vi "GVSView Form Title Frame.vi"() -> ()   [LabVIEW 2013]
uses:
  <vilib>/Utility/miscctls.llb/LVPointTypeDef.ctl
  <vilib>/Utility/miscctls.llb/LVBoundsTypeDef.ctl
  <vilib>/Utility/miscctls.llb/LVPositionTypeDef.ctl
  SubVI/GVSMain Sub Window Global.vi
  GVSView Global.vi
panel:
  in  "pSPRefParent":refnum<vi>
  in  "sClickState":string
  in  "nActiveState":i32
  in  "nIDFrame":i32
  in  "IconRing":u16(ring)
  in  "sViewName":string
  out "TitleName":string caption="Title Name"
  in  "StateOut":bool
  in  "stop":bool
  in  "InActiveClose":bool
  in  "ActiveClose":bool
  in  "bSPResize":bool
  in  "InActiveState":bool
  in  "ActiveStateHalf":bool
  out "SubVI Ref":refnum<vi>
  in  "ActiveState":bool
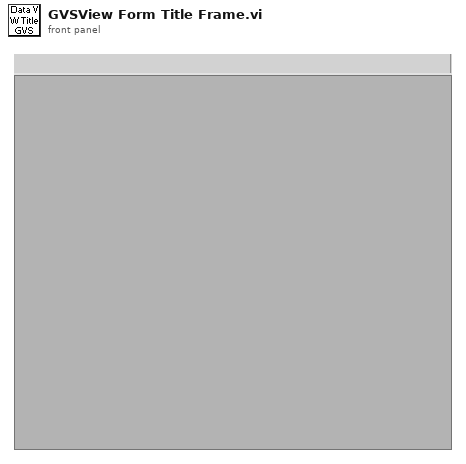
[diagram p1: front panel]
types:
  T1 = typedef "LVPointTypeDef.ctl" = cluster{"Horizontal":i16, "Vertical":i16}
  T2 = typedef "LVBoundsTypeDef.ctl" = cluster{"Width":u32, "Height":u32}
  T3 = typedef "LVPositionTypeDef.ctl" = cluster{"Left":i32, "Top":i32}
  T4 = typedef "LVRectTypeDef.ctl" = cluster{"Left":i16, "Top":i16, "Right":i16, "Bottom":i16}
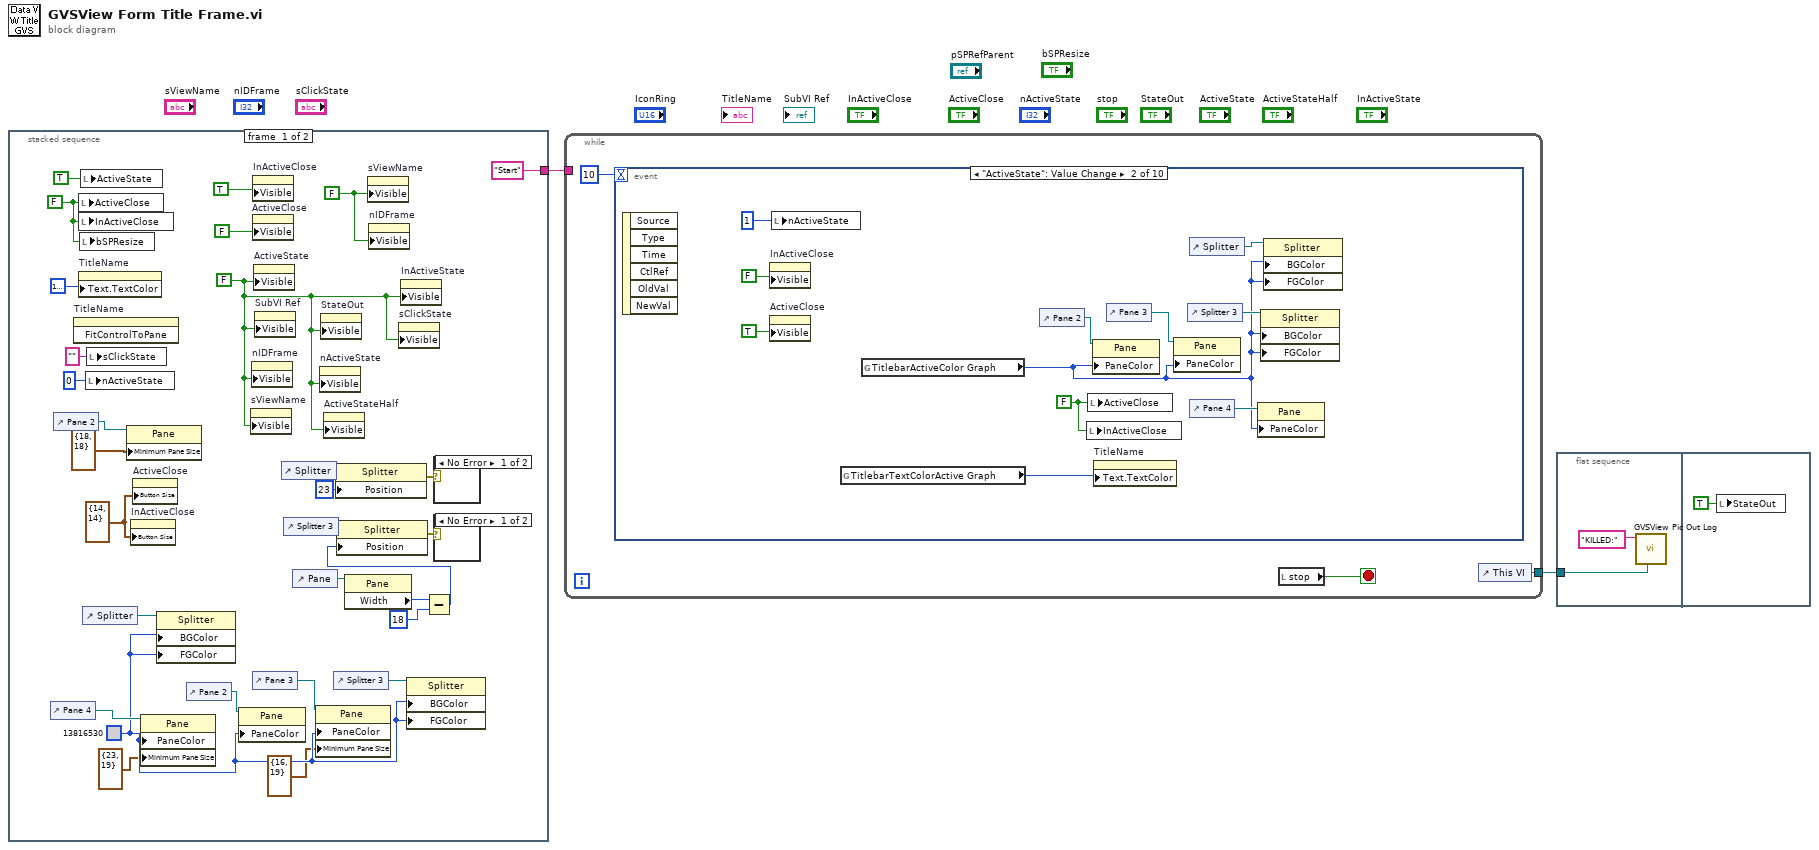
[diagram p0: block diagram]
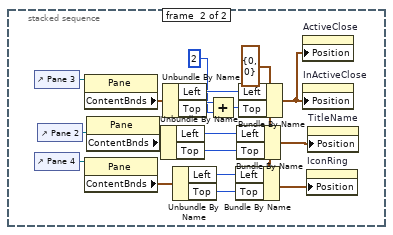
[diagram p4: hidden frame]
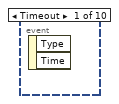
[diagram p5: hidden frame]
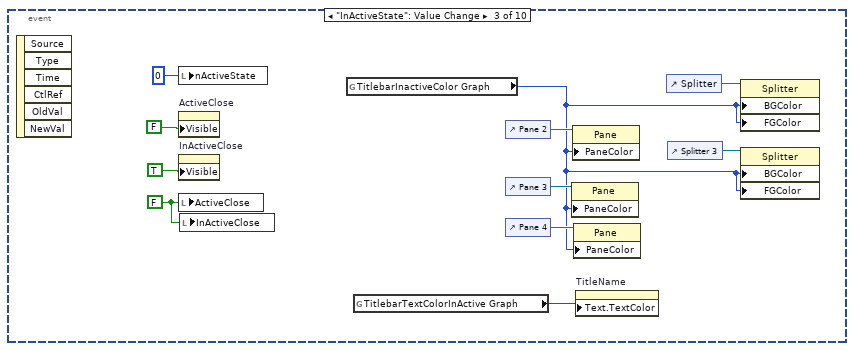
[diagram p6: hidden frame]
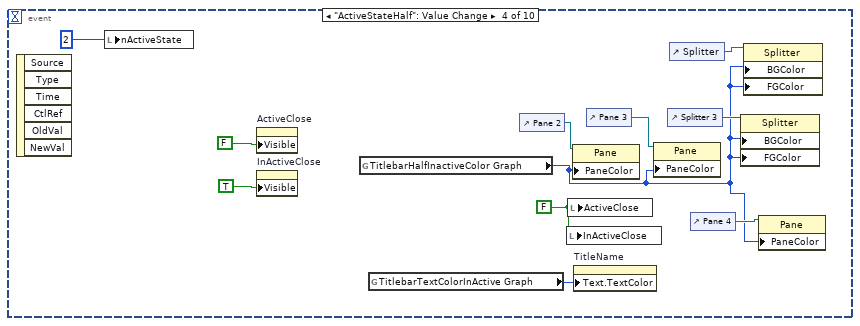
[diagram p7: hidden frame]
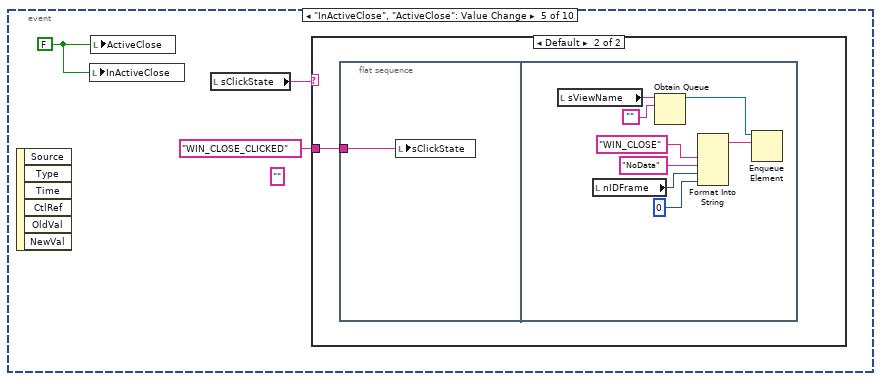
[diagram p8: hidden frame]
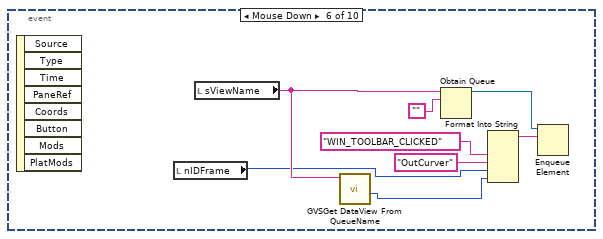
[diagram p10: hidden frame]
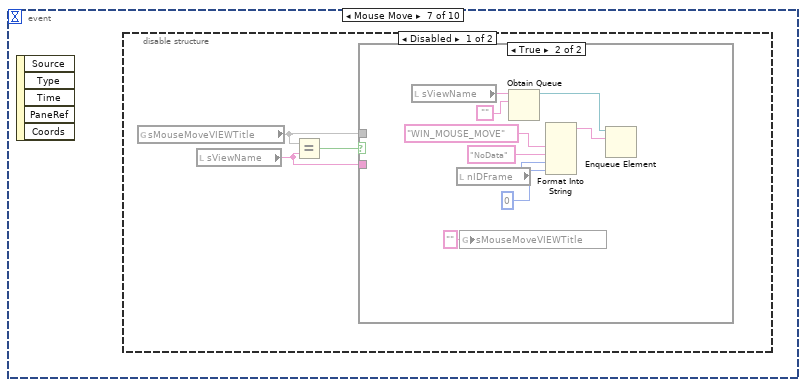
[diagram p11: hidden frame]
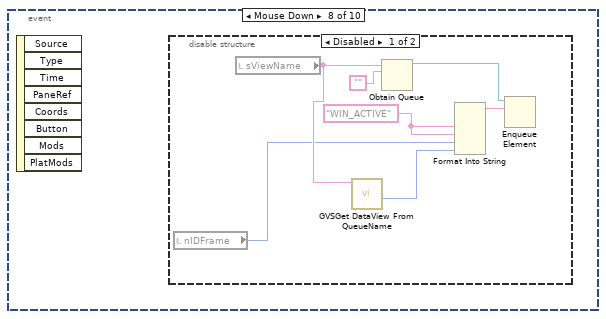
[diagram p14: hidden frame]
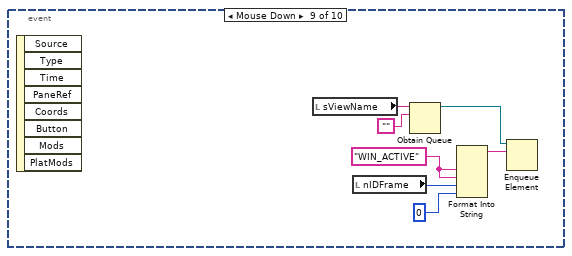
[diagram p16: hidden frame]
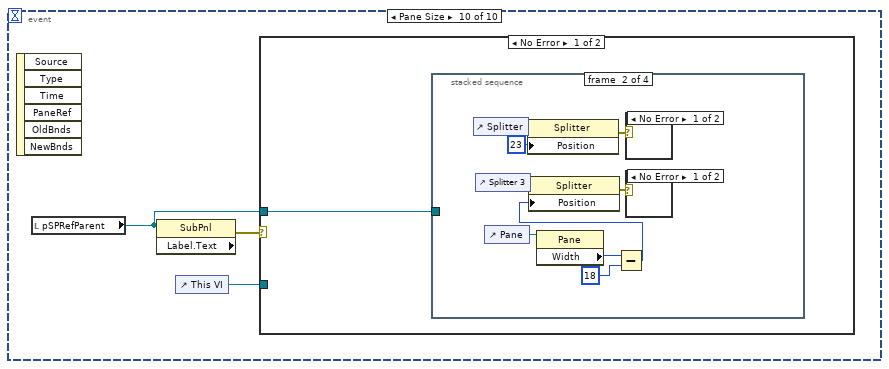
[diagram p17: hidden frame]
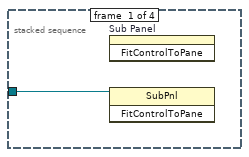
[diagram p18: hidden frame]
diagram:
  n1 = stacked-sequence {
    tunnel: ["Start" _] -> w1
    frame #0 {
      w19 = FALSE ("ToolBar Click")
      w21 = T2 {"Width"=14, "Height"=14} ("Button Size")
      w17 = FALSE ("ToolBar Click")
      w22 = u32 13816530
      w14 = FALSE ("Stop")
      n2 = control-ref of="Pane 4"() -> (w24:refnum<vi>)
      n3 = control-ref of="Pane 2"() -> (w26:refnum<vi>)
      n4 = invoke on="TitleName" class="Str" method="FitControlToPane"() -> ()  [unwired: 3 in, 3 out]
      n5 = local write "ActiveClose"(w14) -> ()
      n6 = local write "InActiveClose"(w14) -> ()
      n7 = property on="TitleName" class="Str"("Text.TextColor"=u32 16777222) -> ()  [unwired: 2 in, 2 out]
      n8 = local write "bSPResize"(w14) -> ()
      n9 = local write "ActiveState"(TRUE ("ActiveState")) -> ()
      n10 = control-ref of="Splitter"() -> (w23:refnum<vi>)
      n11 = local write "nActiveState"(0) -> ()
      n12 = local write "sClickState"("" ("sClickState")) -> ()
      n13 = property class="Pane"(reference=w26, "Minimum Pane Size"=T1 {"Horizontal"=18, "Vertical"=18}) -> ()  [unwired: 1 in, 2 out]
      n14 = property on="InActiveClose" class="Bool (strict)"("Button Size"=w21) -> ()  [unwired: 2 in, 2 out]
      n15 = property on="ActiveClose" class="Bool (strict)"("Button Size"=w21) -> ()  [unwired: 2 in, 2 out]
      n16 = property class="Pane"(reference=w24, "PaneColor"=w22, "Minimum Pane Size"=T1 {"Horizontal"=23, "Vertical"=19}) -> ()  [unwired: 1 in, 2 out]
      n17 = property class="Splitter"(reference=w23, "BGColor"=w22, "FGColor"=w22) -> ()  [unwired: 1 in, 2 out]
      n18 = control-ref of="Pane 2"() -> (w25:refnum<vi>)
      n19 = property class="Pane"(reference=w25, "PaneColor"=w22) -> ()  [unwired: 1 in, 2 out]
      n20 = property on="sViewName" class="Str"("Visible"=w17) -> ()  [unwired: 2 in, 2 out]
      n21 = property on="nIDFrame" class="DigNum (strict)"("Visible"=w17) -> ()  [unwired: 2 in, 2 out]
      n22 = property on="InActiveClose" class="Bool (strict)"("Visible"=TRUE ("ToolBar Click")) -> ()  [unwired: 2 in, 2 out]
      n23 = property on="ActiveClose" class="Bool (strict)"("Visible"=FALSE ("ToolBar Click")) -> ()  [unwired: 2 in, 2 out]
      n24 = control-ref of="Pane 3"() -> (w31:refnum<vi>)
      n25 = property on="ActiveState" class="Bool (strict)"("Visible"=w17) -> ()  [unwired: 2 in, 2 out]
      n26 = property on="SubVI Ref" class="VIRef (strict)"("Visible"=w17) -> ()  [unwired: 2 in, 2 out]
      n27 = control-ref of="Splitter"() -> (w5:refnum<vi>)
      n28 = control-ref of="Splitter 3"() -> (w6:refnum<vi>)
      n29 = control-ref of="Pane"() -> (w8:refnum<vi>)
      n30 = property class="Pane"(reference=w31, "PaneColor"=w22, "Minimum Pane Size"=T1 {"Horizontal"=16, "Vertical"=19}) -> ()  [unwired: 1 in, 2 out]
      n31 = property on="nActiveState" class="DigNum (strict)"("Visible"=w17) -> ()  [unwired: 2 in, 2 out]
      n32 = property on="StateOut" class="Bool (strict)"("Visible"=w17) -> ()  [unwired: 2 in, 2 out]
      n33 = property on="ActiveStateHalf" class="Bool (strict)"("Visible"=w17) -> ()  [unwired: 2 in, 2 out]
      n34 = control-ref of="Splitter 3"() -> (w30:refnum<vi>)
      n35 = property class="Splitter"(reference=w5, "Position"=23 ("Splitter Position")) -> (error out=w11:errorcluster)  [unwired: 1 in, 1 out]
      n36 = property class="Pane"(reference=w8) -> ("Width"=w9:u32)  [unwired: 1 in, 2 out]
      n37 = property on="sViewName" class="Str"("Visible"=w19) -> ()  [unwired: 2 in, 2 out]
      n38 = property on="nIDFrame" class="DigNum (strict)"("Visible"=w19) -> ()  [unwired: 2 in, 2 out]
      n39 = property on="sClickState" class="Str"("Visible"=w17) -> ()  [unwired: 2 in, 2 out]
      n40 = property on="InActiveState" class="Bool (strict)"("Visible"=w17) -> ()  [unwired: 2 in, 2 out]
      n41 = property class="Splitter"(reference=w30, "BGColor"=w22, "FGColor"=w22) -> ()  [unwired: 1 in, 2 out]
      n42 = Subtract(x=w9, y=u32 18) -> (x-y=w10:u32)
      n43 = property class="Splitter"(reference=w6, "Position"=w10) -> (error out=w12:errorcluster)  [unwired: 1 in, 1 out]
      n44 = case shown="No Error" w11 {
        frame No Error {
        }
        frame Error {
        }
      }
      n45 = case shown="No Error" w12 {
        frame No Error {
        }
        frame Error {
        }
      }
    }
    frame #1 {
      w50 = T3 {"Left"=0, "Top"=0} ("Position")
      n46 = control-ref of="Pane 3"() -> (w40:refnum<vi>)
      n47 = control-ref of="Pane 4"() -> (w48:refnum<vi>)
      n48 = control-ref of="Pane 2"() -> (w33:refnum<vi>)
      n49 = property class="Pane"(reference=w40) -> ("ContentBnds"=w39:T4)  [unwired: 1 in, 2 out]
      n50 = property class="Pane"(reference=w48) -> ("ContentBnds"=w46:T4)  [unwired: 1 in, 2 out]
      n51 = property class="Pane"(reference=w33) -> ("ContentBnds"=w43:T4)  [unwired: 1 in, 2 out]
      n52 = Unbundle By Name(w43) -> ("Left"=w42:i16, "Top"=w44:i16)
      n53 = Unbundle By Name(w39) -> ("Left"=w38:i16, "Top"=w36:i16)
      n54 = Unbundle By Name(w46) -> ("Left"=w47:i16, "Top"=w45:i16)
      n55 = Add(x=w36, y=i16 2) -> (x+y=w37:i16)
      n56 = Bundle By Name(cluster=w50, "Left"=w47, "Top"=w45) -> (w49:T3)
      n57 = Bundle By Name(cluster=w50, "Left"=w42, "Top"=w44) -> (w41:T3)
      n58 = Bundle By Name(cluster=w50, "Left"=w38, "Top"=w37) -> (w34:T3)
      n59 = property on="ActiveClose" class="Bool (strict)"("Position"=w34) -> ()  [unwired: 2 in, 2 out]
      n60 = property on="InActiveClose" class="Bool (strict)"("Position"=w34) -> ()  [unwired: 2 in, 2 out]
      n61 = property on="IconRing" class="Ring (strict)"("Position"=w49) -> ()  [unwired: 2 in, 2 out]
      n62 = property on="TitleName" class="Str"("Position"=w41) -> ()  [unwired: 2 in, 2 out]
    }
  }
  n63 = while {
    tunnel: [w52] -> w2
    tunnel: w1 -> [_]
    stop <- w51 stop-if-true
    n64 = event shown="[1] \"ActiveState\": Value Change" {
      selector: _ -> [_ _ _ _ _ _ _ _ _ _]
      dyn-events: _ -> [_ _ _ _ _ _ _ _ _ _]
      timeout: 10 -> [_ _ _ _ _ _ _ _ _ _]
      event Timeout {
        n65 = event-data() -> ()  [unwired: 3 out]
      }
      event "ActiveState": Value Change {
        w62 = FALSE ("Stop")
        n66 = event-data() -> ()  [unwired: 7 out]
        n67 = property on="InActiveClose" class="Bool (strict)"("Visible"=FALSE ("ToolBar Click")) -> ()  [unwired: 2 in, 2 out]
        n68 = property on="ActiveClose" class="Bool (strict)"("Visible"=TRUE ("ToolBar Click")) -> ()  [unwired: 2 in, 2 out]
        n69 = local write "nActiveState"(1) -> ()
        n70 = global read "GVSMain Sub Window Global.vi" "TitlebarTextColorActive Graph"() -> (w55:u32)
        n71 = global read "GVSMain Sub Window Global.vi" "TitlebarActiveColor Graph"() -> (w54:u32)
        n72 = control-ref of="Pane 2"() -> (w61:refnum<vi>)
        n73 = local write "InActiveClose"(w62) -> ()
        n74 = local write "ActiveClose"(w62) -> ()
        n75 = property class="Pane"(reference=w61, "PaneColor"=w54) -> ()  [unwired: 1 in, 2 out]
        n76 = property on="TitleName" class="Str"("Text.TextColor"=w55) -> ()  [unwired: 2 in, 2 out]
        n77 = control-ref of="Pane 3"() -> (w64:refnum<vi>)
        n78 = property class="Pane"(reference=w64, "PaneColor"=w54) -> ()  [unwired: 1 in, 2 out]
        n79 = control-ref of="Splitter 3"() -> (w63:refnum<vi>)
        n80 = control-ref of="Splitter"() -> (w59:refnum<vi>)
        n81 = control-ref of="Pane 4"() -> (w60:refnum<vi>)
        n82 = property class="Pane"(reference=w60, "PaneColor"=w54) -> ()  [unwired: 1 in, 2 out]
        n83 = property class="Splitter"(reference=w63, "BGColor"=w54, "FGColor"=w54) -> ()  [unwired: 1 in, 2 out]
        n84 = property class="Splitter"(reference=w59, "BGColor"=w54, "FGColor"=w54) -> ()  [unwired: 1 in, 2 out]
      }
      event "InActiveState": Value Change {
        w73 = FALSE ("Stop")
        n85 = event-data() -> ()  [unwired: 7 out]
        n86 = local write "nActiveState"(0) -> ()
        n87 = property on="ActiveClose" class="Bool (strict)"("Visible"=FALSE ("ToolBar Click")) -> ()  [unwired: 2 in, 2 out]
        n88 = property on="InActiveClose" class="Bool (strict)"("Visible"=TRUE ("ToolBar Click")) -> ()  [unwired: 2 in, 2 out]
        n89 = local write "ActiveClose"(w73) -> ()
        n90 = local write "InActiveClose"(w73) -> ()
        n91 = global read "GVSMain Sub Window Global.vi" "TitlebarInactiveColor Graph"() -> (w65:u32)
        n92 = global read "GVSMain Sub Window Global.vi" "TitlebarTextColorInActive Graph"() -> (w66:u32)
        n93 = control-ref of="Pane 2"() -> (w72:refnum<vi>)
        n94 = control-ref of="Pane 3"() -> (w75:refnum<vi>)
        n95 = control-ref of="Pane 4"() -> (w71:refnum<vi>)
        n96 = property class="Pane"(reference=w75, "PaneColor"=w65) -> ()  [unwired: 1 in, 2 out]
        n97 = property class="Pane"(reference=w72, "PaneColor"=w65) -> ()  [unwired: 1 in, 2 out]
        n98 = property class="Pane"(reference=w71, "PaneColor"=w65) -> ()  [unwired: 1 in, 2 out]
        n99 = property on="TitleName" class="Str"("Text.TextColor"=w66) -> ()  [unwired: 2 in, 2 out]
        n100 = control-ref of="Splitter"() -> (w70:refnum<vi>)
        n101 = control-ref of="Splitter 3"() -> (w74:refnum<vi>)
        n102 = property class="Splitter"(reference=w70, "BGColor"=w65, "FGColor"=w65) -> ()  [unwired: 1 in, 2 out]
        n103 = property class="Splitter"(reference=w74, "BGColor"=w65, "FGColor"=w65) -> ()  [unwired: 1 in, 2 out]
      }
      event "ActiveStateHalf": Value Change {
        w84 = FALSE ("Stop")
        n104 = event-data() -> ()  [unwired: 7 out]
        n105 = local write "nActiveState"(2) -> ()
        n106 = property on="ActiveClose" class="Bool (strict)"("Visible"=FALSE ("ToolBar Click")) -> ()  [unwired: 2 in, 2 out]
        n107 = property on="InActiveClose" class="Bool (strict)"("Visible"=TRUE ("ToolBar Click")) -> ()  [unwired: 2 in, 2 out]
        n108 = global read "GVSMain Sub Window Global.vi" "TitlebarHalfInactiveColor Graph"() -> (w77:u32)
        n109 = global read "GVSMain Sub Window Global.vi" "TitlebarTextColorInActive Graph"() -> (w76:u32)
        n110 = control-ref of="Pane 2"() -> (w83:refnum<vi>)
        n111 = local write "InActiveClose"(w84) -> ()
        n112 = local write "ActiveClose"(w84) -> ()
        n113 = property class="Pane"(reference=w83, "PaneColor"=w77) -> ()  [unwired: 1 in, 2 out]
        n114 = property on="TitleName" class="Str"("Text.TextColor"=w76) -> ()  [unwired: 2 in, 2 out]
        n115 = control-ref of="Pane 3"() -> (w86:refnum<vi>)
        n116 = property class="Pane"(reference=w86, "PaneColor"=w77) -> ()  [unwired: 1 in, 2 out]
        n117 = control-ref of="Splitter 3"() -> (w85:refnum<vi>)
        n118 = control-ref of="Splitter"() -> (w81:refnum<vi>)
        n119 = control-ref of="Pane 4"() -> (w82:refnum<vi>)
        n120 = property class="Splitter"(reference=w85, "BGColor"=w77, "FGColor"=w77) -> ()  [unwired: 1 in, 2 out]
        n121 = property class="Splitter"(reference=w81, "BGColor"=w77, "FGColor"=w77) -> ()  [unwired: 1 in, 2 out]
        n122 = property class="Pane"(reference=w82, "PaneColor"=w77) -> ()  [unwired: 1 in, 2 out]
      }
      event "InActiveClose", "ActiveClose": Value Change {
        w87 = FALSE ("Stop")
        (unwired) "" ("sData")
        n123 = event-data() -> ()  [unwired: 7 out]
        n124 = local write "InActiveClose"(w87) -> ()
        n125 = local write "ActiveClose"(w87) -> ()
        n126 = local read "sClickState"() -> (w89:string)
        n127 = case shown="Default" w89 {
          tunnel: "WIN_CLOSE_CLICKED" ("sData") -> [_ w90]
          frame "WIN_CLOSE_CLICKED" {
          }
          frame Default {
            n128 = flat-sequence {
              tunnel: w90 -> [w91]
              frame #0 {
                n129 = local write "sClickState"(w91) -> ()
              }
              frame #1 {
                n130 = local read "sViewName"() -> (w94:string)
                n131 = local read "nIDFrame"() -> (w96:i32)
                n132 = Obtain Queue(name (unnamed)=w94, element data type="") -> (queue out=w93:refnum<queue>)  [unwired: 3 in, 2 out]
                n133 = Format Into String("WIN_CLOSE" ("input 1"), "NoData" ("input 2"), w96, 0 ("input 3")) -> (resulting string=w92:string)  [unwired: 3 in, 1 out]
                n134 = Enqueue Element(queue=w93, element=w92) -> ()  [unwired: 1 in, 4 out]
              }
            }
          }
        }
      }
      event Mouse Down {
        n135 = event-data() -> ()  [unwired: 9 out]
        n136 = local read "nIDFrame"() -> (w100:i32)
        n137 = local read "sViewName"() -> (w102:string)
        n138 = call "GVSGet DataView From QueueName.vi"("DataView QueueName"=w102) -> ("DataView Idx out"=w101:i32)  [unwired: 8 in, 2 out]
        n139 = Obtain Queue(name (unnamed)=w102, element data type="") -> (queue out=w105:refnum<queue>)  [unwired: 3 in, 2 out]
        n140 = Format Into String("WIN_TOOLBAR_CLICKED" ("input 1"), "OutCurver" ("input 2"), w100, w101) -> (resulting string=w103:string)  [unwired: 3 in, 1 out]
        n141 = Enqueue Element(queue=w105, element=w103) -> ()  [unwired: 1 in, 4 out]
      }
      event Mouse Move {
        n142 = event-data() -> ()  [unwired: 6 out]
        n143 = disable-structure shown="Disabled" {
          frame Disabled {
            n144 = global read "GVSView Global.vi" "sMouseMoveVIEWTitle"() -> (w109)
            n145 = local read "sViewName"() -> (w108:string)
            n146 = Equal?(x=w109, y=w108) -> (x = y?=w110:bool)
            n147 = case shown="True" w110 {
              tunnel: w109 -> [_ _]
              tunnel: w108 -> [_ _]
              frame False {
              }
              frame True {
                n148 = local read "sViewName"() -> (w113:string)
                n149 = local read "nIDFrame"() -> (w116:i32)
                n150 = global write "GVSView Global.vi" "sMouseMoveVIEWTitle"("" ("sMouseMoveVIEWTitle")) -> ()
                n151 = Obtain Queue(name (unnamed)=w113, element data type="") -> (queue out=w115:refnum<queue>)  [unwired: 3 in, 2 out]
                n152 = Format Into String("WIN_MOUSE_MOVE" ("input 1"), "NoData" ("input 2"), w116, 0 ("input 3")) -> (resulting string=w112:string)  [unwired: 3 in, 1 out]
                n153 = Enqueue Element(queue=w115, element=w112) -> ()  [unwired: 1 in, 4 out]
              }
            }
          }
          frame Enabled {
          }
        }
      }
      event Mouse Down {
        n154 = event-data() -> ()  [unwired: 9 out]
        n155 = disable-structure shown="Disabled" {
          frame Disabled {
            w123 = "WIN_ACTIVE" ("input 1")
            n156 = local read "nIDFrame"() -> (w120:i32)
            n157 = local read "sViewName"() -> (w122:string)
            n158 = call "GVSGet DataView From QueueName.vi"("DataView QueueName"=w122) -> ("DataView Idx out"=w121:i32)  [unwired: 8 in, 2 out]
            n159 = Obtain Queue(name (unnamed)=w122, element data type="") -> (queue out=w126:refnum<queue>)  [unwired: 3 in, 2 out]
            n160 = Format Into String(w123, w123, w120, w121) -> (resulting string=w124:string)  [unwired: 3 in, 1 out]
            n161 = Enqueue Element(queue=w126, element=w124) -> ()  [unwired: 1 in, 4 out]
          }
          frame Enabled {
          }
        }
      }
      event Mouse Down {
        w127 = "WIN_ACTIVE" ("input 1")
        n162 = event-data() -> ()  [unwired: 9 out]
        n163 = local read "sViewName"() -> (w129:string)
        n164 = local read "nIDFrame"() -> (w132:i32)
        n165 = Obtain Queue(name (unnamed)=w129, element data type="") -> (queue out=w131:refnum<queue>)  [unwired: 3 in, 2 out]
        n166 = Format Into String(w127, w127, w132, 0 ("input 3")) -> (resulting string=w128:string)  [unwired: 3 in, 1 out]
        n167 = Enqueue Element(queue=w131, element=w128) -> ()  [unwired: 1 in, 4 out]
      }
      event Pane Size {
        n168 = event-data() -> ()  [unwired: 7 out]
        n169 = local read "pSPRefParent"() -> (w135:refnum<vi>)
        n170 = property class="SubPnl" props=["Label", "Text"](reference=w135) -> (error out=w136:errorcluster)  [unwired: 1 in, 2 out]
        n171 = control-ref of="This VI"() -> (w134:refnum<vi>)
        n172 = case shown="No Error" w136 {
          tunnel: w135 -> [w137 _]
          tunnel: w134 -> [_ _]
          frame No Error {
            n173 = stacked-sequence {
              tunnel: w137 -> [w138 _ _ _]
              frame #0 {
                n174 = invoke on="Sub Panel" class="SubPnl" method="FitControlToPane"() -> ()  [unwired: 3 in, 3 out]
                n175 = invoke class="SubPnl" method="FitControlToPane"(reference=w138) -> ()  [unwired: 2 in, 3 out]
              }
              frame #1 {
                n176 = control-ref of="Splitter"() -> (w139:refnum<vi>)
                n177 = control-ref of="Splitter 3"() -> (w140:refnum<vi>)
                n178 = control-ref of="Pane"() -> (w142:refnum<vi>)
                n179 = property class="Splitter"(reference=w139, "Position"=23 ("Splitter Position")) -> (error out=w145:errorcluster)  [unwired: 1 in, 1 out]
                n180 = property class="Pane"(reference=w142) -> ("Width"=w143:u32)  [unwired: 1 in, 2 out]
                n181 = Subtract(x=w143, y=u32 18) -> (x-y=w144:u32)
                n182 = property class="Splitter"(reference=w140, "Position"=w144) -> (error out=w146:errorcluster)  [unwired: 1 in, 1 out]
                n183 = case shown="No Error" w145 {
                  frame No Error {
                  }
                  frame Error {
                  }
                }
                n184 = case shown="No Error" w146 {
                  frame No Error {
                  }
                  frame Error {
                  }
                }
              }
              frame #2 {
                w148 = T3 {"Left"=0, "Top"=0} ("Position")
                n185 = control-ref of="Pane 3"() -> (w158:refnum<vi>)
                n186 = control-ref of="Pane 4"() -> (w150:refnum<vi>)
                n187 = control-ref of="Pane 2"() -> (w165:refnum<vi>)
                n188 = property class="Pane"(reference=w158) -> ("ContentBnds"=w159:T4)  [unwired: 1 in, 2 out]
                n189 = property class="Pane"(reference=w150) -> ("ContentBnds"=w152:T4)  [unwired: 1 in, 2 out]
                n190 = property class="Pane"(reference=w165) -> ("ContentBnds"=w155:T4)  [unwired: 1 in, 2 out]
                n191 = Unbundle By Name(w155) -> ("Left"=w156:i16, "Top"=w154:i16)
                n192 = Unbundle By Name(w159) -> ("Left"=w160:i16, "Top"=w162:i16)
                n193 = Unbundle By Name(w152) -> ("Left"=w151:i16, "Top"=w153:i16)
                n194 = Add(x=w162, y=i16 2) -> (x+y=w161:i16)
                n195 = Bundle By Name(cluster=w148, "Left"=w151, "Top"=w153) -> (w149:T3)
                n196 = Bundle By Name(cluster=w148, "Left"=w156, "Top"=w154) -> (w157:T3)
                n197 = Bundle By Name(cluster=w148, "Left"=w160, "Top"=w161) -> (w164:T3)
                n198 = property on="ActiveClose" class="Bool (strict)"("Position"=w164) -> ()  [unwired: 2 in, 2 out]
                n199 = property on="InActiveClose" class="Bool (strict)"("Position"=w164) -> ()  [unwired: 2 in, 2 out]
                n200 = property on="IconRing" class="Ring (strict)"("Position"=w149) -> ()  [unwired: 2 in, 2 out]
                n201 = property on="TitleName" class="Str"("Position"=w157) -> ()  [unwired: 2 in, 2 out]
              }
              frame #3 {
                n202 = local write "bSPResize"(TRUE ("bSPResize")) -> ()
              }
            }
          }
          frame Error {
            n203 = local write "bSPResize"(TRUE ("bSPResize")) -> ()
          }
        }
      }
    }
    n204 = local read "stop"() -> (w51:bool)
    n205 = control-ref of="This VI"() -> (w52:refnum<vi>)
  }
  n206 = flat-sequence {
    tunnel: w2 -> [w169]
    frame #0 {
      n207 = call "GVSView Pic Out Log.vi"("vi reference"=w169, "sData"="KILLED:") -> ()  [unwired: 10 in]
    }
    frame #1 {
      n208 = local write "StateOut"(TRUE ("StateOut")) -> ()
    }
  }
